vi "Get Firmware Version.vi"() -> (3 "Firmware Version String":string)   [LabVIEW 2015, in "Tool Cfg.lvlib"]
uses:
  Tool Cfg.lvlib
  ConfigGLOB.vi
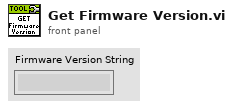
[diagram p1: front panel]
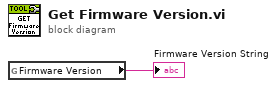
[diagram p0: block diagram]
diagram:
  n1 = global read "ConfigGLOB.vi" "Firmware Version"() -> (→"Firmware Version String":string)
